vi "Auton All Stop.vi"(8 "Refnum in":refnum<k33>) -> (0 "Refnum out":refnum<k33>)   [LabVIEW 2014]
uses:
  TeleopCmd.ctl
  CmdFlag.ctl
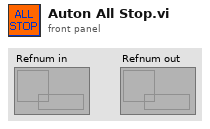
[diagram p1: front panel]
types:
  T1 = typedef "TeleopCmd.ctl" = cluster{"CmdFlag":T2, "throttle":dbl, "turn":dbl, "Override":bool, "Strafe":dbl, "MotorPwrMax":u8, "Time":u32}
  T2 = typedef "CmdFlag.ctl" = enum16{"noop", "logflag", "suspend", "resume"}
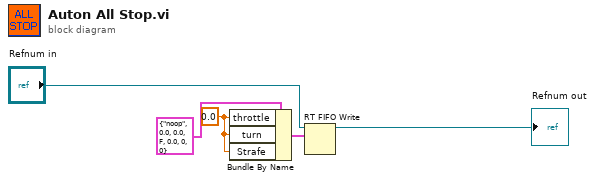
[diagram p0: block diagram]
diagram:
  w4 = 0.0 ("throttle")
  n1 = Bundle By Name(cluster=T1 {"CmdFlag"=enum."noop", "throttle"=0.0, "turn"=0.0, "Override"=FALSE, "Strafe"=0.0, "MotorPwrMax"=0, "Time"=0} ("Cluster"), "throttle"=w4, "turn"=w4, "Strafe"=w4) -> (w2:T1)
  n2 = RT FIFO Write(0:"Refnum in", 1:w2) -> (8:→"Refnum out":refnum<k33>)  [unwired: 3 in, 3 out]
